vi "getLowValue.vi"(8 "error in (no error)":errorcluster, 11 "IRange in":refnum<class "IRange.lvclass">) -> (0 "error out":errorcluster, 2 "Low Value out":i64, 3 "IRange out":refnum<class "IRange.lvclass">)   [LabVIEW 2022 SP3, in "openDAQ.lvlib" / "daqCoreTypes.lvlib" / "IRange.lvclass"]
uses:
  <instrlib>/openDAQ/Public/Classes/daqCoreTypes/IRange/IRange.lvclass
  <instrlib>/openDAQ/Public/Classes/daqCoreTypes/IRange/IRange.lvclass/IRange.ctl
  <instrlib>/openDAQ/Public/Classes/daqCoreTypes/INumber/INumber.lvclass
  <instrlib>/openDAQ/Binaries/Windows/x86/copendaq32.dll
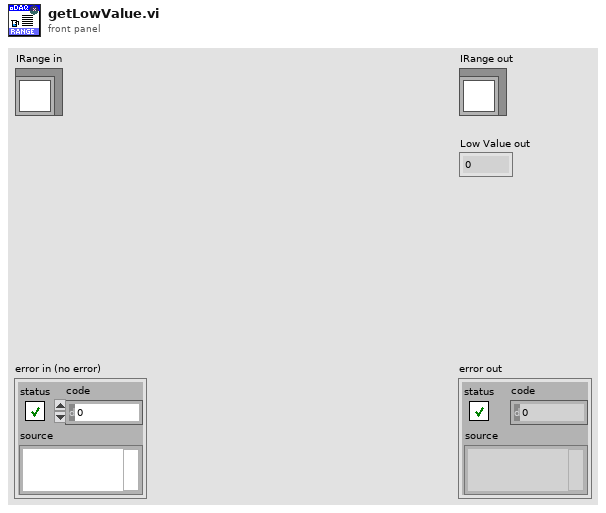
[diagram p1: front panel]
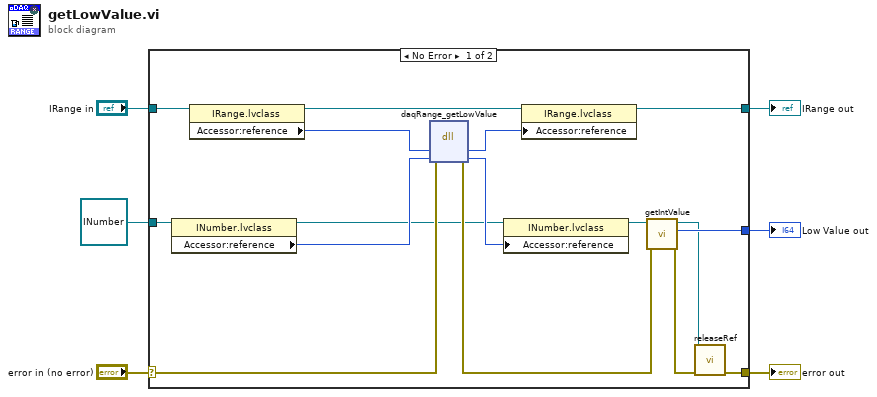
[diagram p0: block diagram]
diagram:
  n1 = case shown="No Error" "error in (no error)" {
    selector: "error in (no error)" -> [w18 w24]
    tunnel: [w9 w24] -> w5
    tunnel: [w16 w23] -> w3
    tunnel: "IRange in" -> [w19 w23]
    tunnel: refnum<class "INumber.lvclass"> refnum ("openDAQ.lvlib:daqCoreTypes.lvlib:INumber.lvclass") -> [w13 _]
    tunnel: [w20 _] -> w1
    frame No Error {
      n2 = property class="INumber.lvclass"(reference=w13) -> (reference out=w11:refnum<class "INumber.lvclass">, "Accessor:reference"=w12:i64)  [unwired: 1 in, 1 out]
      n3 = property class="IRange.lvclass"(reference=w19) -> (reference out=w17:refnum<class "IRange.lvclass">, "Accessor:reference"=w15:i64)  [unwired: 1 in, 1 out]
      n4 = dll-call lib="C:/Program Files (x86)/National Instruments/LabVIEW 2022/instr.lib/openDAQ/Binaries/Windows/x86/copendaq*.*" fn="daqRange_getLowValue"(error in=w18, "range"=w15, "lowValue"=w12) -> (error out=w21:errorcluster, "range"=w14:i64, "lowValue"=w22:i64)  [unwired: 3 in, 1 out]
      n5 = property class="INumber.lvclass"(reference=w11, "Accessor:reference"=w22) -> (reference out=w10:refnum<class "INumber.lvclass">)  [unwired: 1 in, 1 out]
      n6 = property class="IRange.lvclass"(reference=w17, "Accessor:reference"=w14) -> (reference out=w16:refnum<class "IRange.lvclass">)  [unwired: 1 in, 1 out]
      n7 = call <instrlib>:"getIntValue.vi"("error in (no error)"=w21, "INumber in"=w10) -> ("error out"=w8:errorcluster, "Int Value out"=w20:i64, "INumber out"=w7:refnum<class "INumber.lvclass">)  [unwired: 7 in]
      n8 = call-dynamic "releaseRef.vi"("error in (no error)"=w8, "IBaseObject in"=w7) -> ("error out"=w9:errorcluster)  [unwired: 9 in]
    }
    frame Error {
    }
  }
  "error out" <- w5
  "IRange out" <- w3
  "Low Value out" <- w1
